vi "Set ListObj.vi"(8 "error in (no error)":errorcluster, 10 "List Object":refnum<class "List.lvclass">, 11 "StringList in":refnum<class "StringList.lvclass">) -> (0 "error out":errorcluster, 3 "StringList out":refnum<class "StringList.lvclass">)   [LabVIEW 2017, in "LapDog.Collections.v0.Lists.Interfaces.lvlib" / "StringList.lvclass"]
uses:
  StringList.lvclass
  Lists/List/List.lvclass
  StringList.lvclass/StringList.ctl
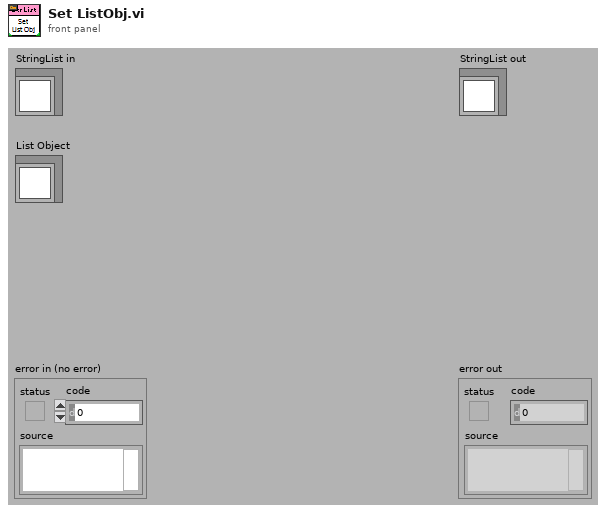
[diagram p1: front panel]
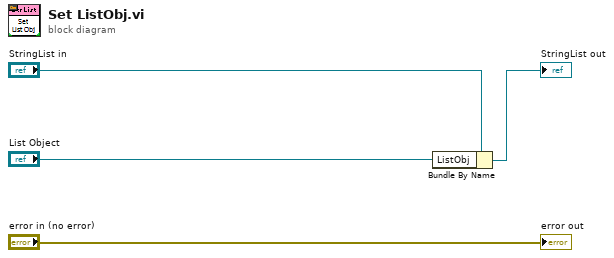
[diagram p0: block diagram]
diagram:
  n1 = Bundle By Name(cluster="StringList in", "ListObj"="List Object") -> (→"StringList out":refnum<class "StringList.lvclass">)
  "error out" <- "error in (no error)"
